vi "Property Node (XNET TCP Socket).vi"   [LabVIEW 2018]
doc: "Provides properties that can be used with the XNET TCP Socket VIs."
uses:
  <resource>/objmgr/xnet.rc
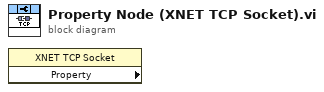
[diagram p0: block diagram]
diagram:
  n1 = property class="XNET TCP Socket" props=[]() -> ()  [unwired: 2 in, 3 out]
